vi "Write Key Value Double.vi"(7 "Section Name":string, 8 "error in (no error)":errorcluster, 9 "Value":dbl, 10 "Key Name":string, 11 "Interface in":refnum<class "Interface.lvclass">) -> (0 "error out":errorcluster, 2 "found":bool, 3 "Interface out":refnum<class "Interface.lvclass">)   [LabVIEW 2016, in "Configuration.lvlib" / "Interface.lvclass"]
doc: "Write double key value."
uses:
  Interface.lvclass
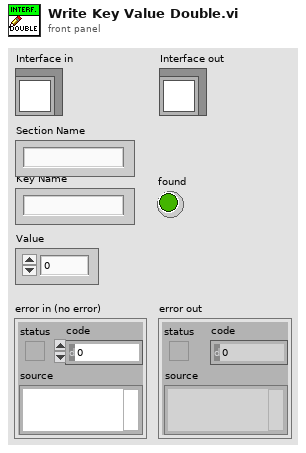
[diagram p1: front panel]
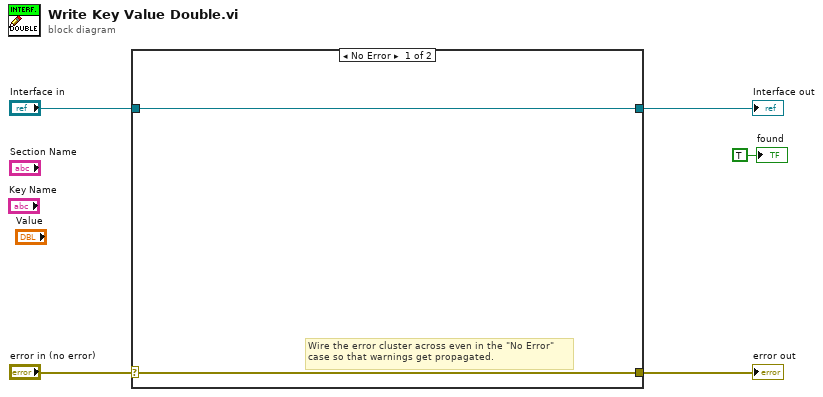
[diagram p0: block diagram]
diagram:
  n1 = case shown="No Error" "error in (no error)" {
    selector: "error in (no error)" -> [w7 w9]
    tunnel: [w7 w9] -> w4
    tunnel: [w6 w8] -> w2
    tunnel: "Interface in" -> [w6 w8]
    frame No Error {
      # "Wire the error cluster across even in the \"No Error\"\ncase so that warnings get propagated."
    }
    frame Error {
    }
  }
  "error out" <- w4
  "Interface out" <- w2
  "found" <- TRUE ("found")
